vi "Nexteer connect.vi"(6 "error in":errorcluster, 8 "MaxRead":i32, 9 "Channel in":u16 format="%.0x") -> (0 "error out":errorcluster, 1 "Messages":T1(array[cluster]), 2 "Pass":bool, 3 "Channel out":u16)   [LabVIEW 2023]
uses:
  Communication/PCAN2023/PCAN API.lvlib
  0453edcd-7fdf-4f9d-9433-77afa8cb6083.vi
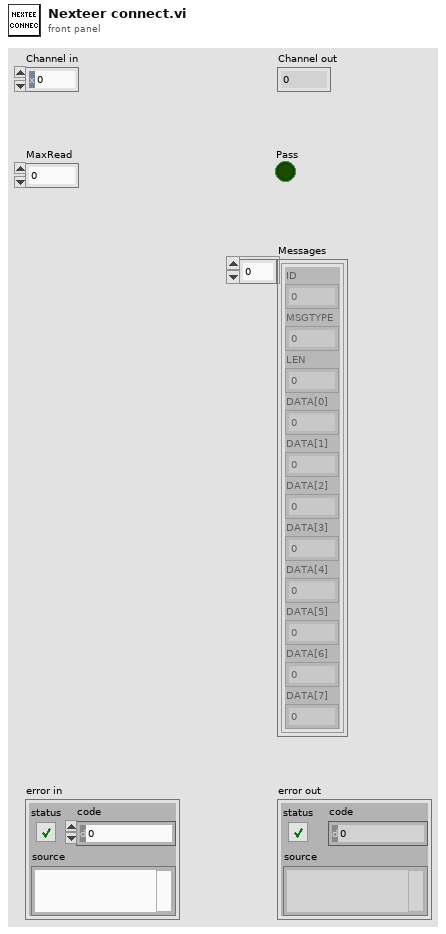
[diagram p1: front panel]
types:
  T1 = cluster{"ID":u32, "MSGTYPE":u8, "LEN":u8, "DATA[0]":u8, "DATA[1]":u8, "DATA[2]":u8, "DATA[3]":u8, "DATA[4]":u8, "DATA[5]":u8, "DATA[6]":u8, "DATA[7]":u8}[]
  T2 = cluster{"ID":u32, "MSGTYPE":u8, "LEN":u8, "DATA[0]":u8, "DATA[1]":u8, "DATA[2]":u8, "DATA[3]":u8, "DATA[4]":u8, "DATA[5]":u8, "DATA[6]":u8, "DATA[7]":u8}
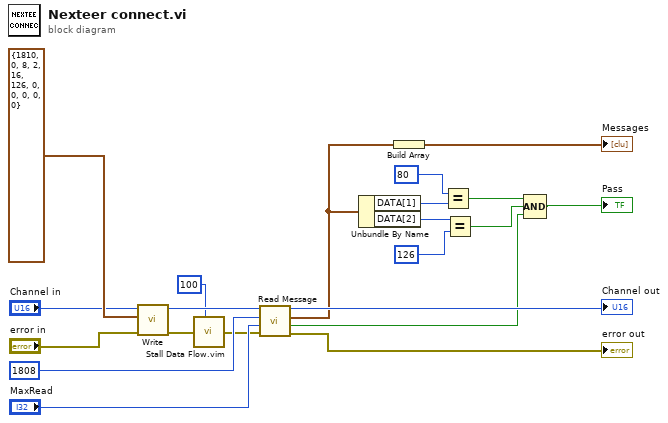
[diagram p0: block diagram]
diagram:
  n1 = call "Write.vi"("error in"="error in", "MessageBuffer"=T2 {"ID"=1810, "MSGTYPE"=0, "LEN"=8, "DATA[0]"=2, "DATA[1]"=16, "DATA[2]"=126, "DATA[3]"=0, "DATA[4]"=0, "DATA[5]"=0, "DATA[6]"=0, "DATA[7]"=0}, "Channel"="Channel in") -> ("error out"=w8:errorcluster, "Channel out"=w10:u16)  [unwired: 5 in, 2 out]
  n2 = call "Stall Data Flow.vim"("value in"=w8, "milliseconds to wait"=u32 100) -> ("value out"=w2:errorcluster)  [unwired: 1 out]
  n3 = call "Read Message.vi"("error in"=w2, "MaxRead"="MaxRead", "ID"=u32 1808, "Channel in"=w10) -> ("error out"=→"error out":errorcluster, "Passed"=w3:bool, "Last Message"=w4:T2, "Channel out"=→"Channel out":u16)  [unwired: 3 in, 1 out]
  n4 = Unbundle By Name(w4) -> ("DATA[1]"=w18:u8, "DATA[2]"=w16:u8)
  n5 = Build Array(w4) -> (→"Messages":T1)
  n6 = Equal?(x=u8 80, y=w18) -> (x = y?=w14:bool)
  n7 = Equal?(x=w16, y=u8 126 ("x")) -> (x = y?=w13:bool)
  n8 = Compound Arithmetic op=AND(w14, w13, w3) -> (→"Pass":bool)
